vi "pickKeeperRobots.vi"(8 "error in (no error)":errorcluster, 11 "Game in":refnum<class "Game.lvclass">) -> (0 "error out":errorcluster, 3 "Game out":refnum<class "Game.lvclass">)   [LabVIEW 2023, in "Game.lvclass"]
uses:
  Game.lvclass
  Game.lvclass/Game.ctl
  Team_class/Team.lvclass/Team.ctl
  Referee_class/Referee.lvclass/Referee.ctl
  Playbook_class/Playbook.lvclass/Playbook.ctl
  TestPlay_class/TestPlay.lvclass/TestPlay.ctl
  Robot_class/roles.ctl
  Robot_class/Robot.lvclass/Robot.ctl
  Role_class/Role.lvclass/Role.ctl
  HaltPlay_class/HaltPlay.lvclass/HaltPlay.ctl
  TimeoutPlay_class/TimeoutPlay.lvclass/TimeoutPlay.ctl
  ZigZagPlay_class/ZigZagPlay.lvclass/ZigZagPlay.ctl
  Role_class/Write RobotRef.vi
  TestPlay_class/Read Roles.vi
  Robot_class/Write role.vi
  TestPlay_class/Write Roles.vi
  Playbook_class/Write keeper_plays.vi
  Playbook_class/Read keeper_plays.vi
  TestPlay_class/Read NumberOfRobots.vi
  HaltPlay_class/Read Roles.vi
  HaltPlay_class/Write Roles.vi
  HaltPlay_class/Read NumberOfRobots.vi
  TimeoutPlay_class/Read Roles.vi
  TimeoutPlay_class/Write Roles.vi
  ZigZagPlay_class/Read Roles.vi
  ZigZagPlay_class/Write Roles.vi
  Read KeeperTeam.vi
  Read AllyRef.vi
  Read Referee.vi
  Read TestMode IDs.vi
  Referee_class/Read our_goalie_id.vi
  Team_class/Read KeeperPlay.vi
  Team_class/Read RobotRef.vi
  Team_class/Write RobotRef.vi
  Write KeeperTeam.vi
  Ally_class/Ally.lvclass
  C:/Users/roboi/Downloads/VSS_AI-Larc2023/Team_class/Team.lvclass
  TestRole_class/TestRole.lvclass
  C:/Users/roboi/Downloads/VSS_AI-Larc2023/Role_class/Role.lvclass
  HaltRole_class/HaltRole.lvclass
  TimeoutRole_class/TimeoutRole.lvclass
  KeeperRole_class/KeeperRole.lvclass
  ZigZagRole_class/ZigZagRole.lvclass
  Referee_class/Referee.lvclass
  Playbook_class/Playbook.lvclass
  Robot_class/Robot.lvclass
  Play_class/Play.lvclass
  TestPlay_class/TestPlay.lvclass
  HaltPlay_class/HaltPlay.lvclass
  KeeperPlay_class/KeeperPlay.lvclass
  TimeoutPlay_class/TimeoutPlay.lvclass
  ZigZagPlay_class/ZigZagPlay.lvclass
  GoToPlay_class/GoToPlay.lvclass
  Role_class/Role.lvclass
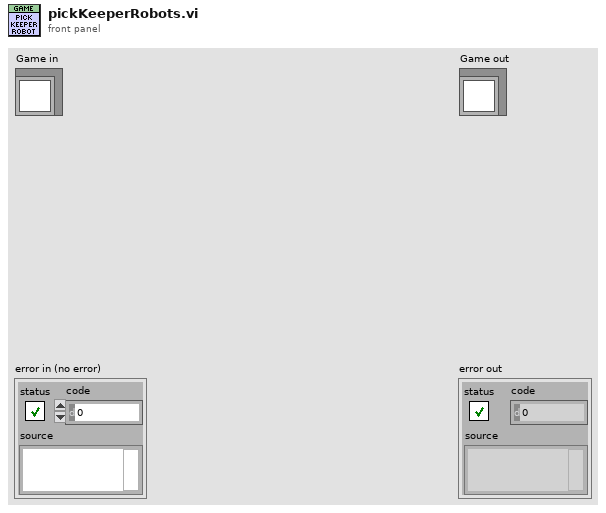
[diagram p1: front panel]
types:
  T1 = typedef "roles.ctl" = enum16{"BallChallengerAttackerVSS", "NormalAttackerVSS", "AttackerAimGoalVSS", "DefenderAreaVSS", "KeeperVSS", "Tabler", "TableFinalizer", "PrepareRollToPassRoller", "PrepareRollToPassReceiver", "SimplePassRoll", "SimplePassRollReceiver", "PenaltyDefense", "PreparePassReceiver 2", "PreparePassReceiver 1", "PassObserver", "Timeout", "Goto", "ZigZag", "None", "BallOutOfField", "DefenderArea", "Duelist", "AttackerStop", "FollowAttacker", "KeeperRole", "KickPenalty", "AttackerAimGoal", "AttackerBlock", "Marker", "Halt", "Shoot", "PassKicker", "PassReceiver", "TestRole", "PenaltyAttacker"}
  T2 = typedef "KeeperPlay.ctl" = enum16{"ZigZag", "Goto", "NormalGame", "KeeperPlay", "Halt", "Timeout", "PenaltyEnemy", "TestPlay"}
  T3 = typedef "keeper_plays.ctl" = cluster{"Play":refnum<class "Play.lvclass">, "TestPlay":refnum<class "TestPlay.lvclass">, "HaltPlay":refnum<class "HaltPlay.lvclass">, "KeeperPlay":refnum<class "KeeperPlay.lvclass">, "TimeoutPlay":refnum<class "TimeoutPlay.lvclass">, "ZigZagPlay":refnum<class "ZigZagPlay.lvclass">, "GoToPlay":refnum<class "GoToPlay.lvclass">}
  T4 = cluster{"TestRole 1":refnum<class "TestRole.lvclass">, "Role":refnum<class "Role.lvclass">, "TestRole 2":refnum<class "TestRole.lvclass">, "TestRole 3":refnum<class "TestRole.lvclass">}
  T5 = cluster{"HaltRole 1":refnum<class "HaltRole.lvclass">, "HaltRole 2":refnum<class "HaltRole.lvclass">, "HaltRole 3":refnum<class "HaltRole.lvclass">, "HaltRole 4":refnum<class "HaltRole.lvclass">, "HaltRole 5":refnum<class "HaltRole.lvclass">, "HaltRole 6":refnum<class "HaltRole.lvclass">}
  T6 = cluster{"TimeoutRole 1":refnum<class "TimeoutRole.lvclass">, "TimeoutRole 2":refnum<class "TimeoutRole.lvclass">, "TimeoutRole 3":refnum<class "TimeoutRole.lvclass">, "TimeoutRole 4":refnum<class "TimeoutRole.lvclass">, "TimeoutRole 5":refnum<class "TimeoutRole.lvclass">, "TimeoutRole 6":refnum<class "TimeoutRole.lvclass">}
  T7 = cluster{"KeeperRole":refnum<class "KeeperRole.lvclass">}
  T8 = cluster{"ZigZagRole":refnum<class "ZigZagRole.lvclass">}
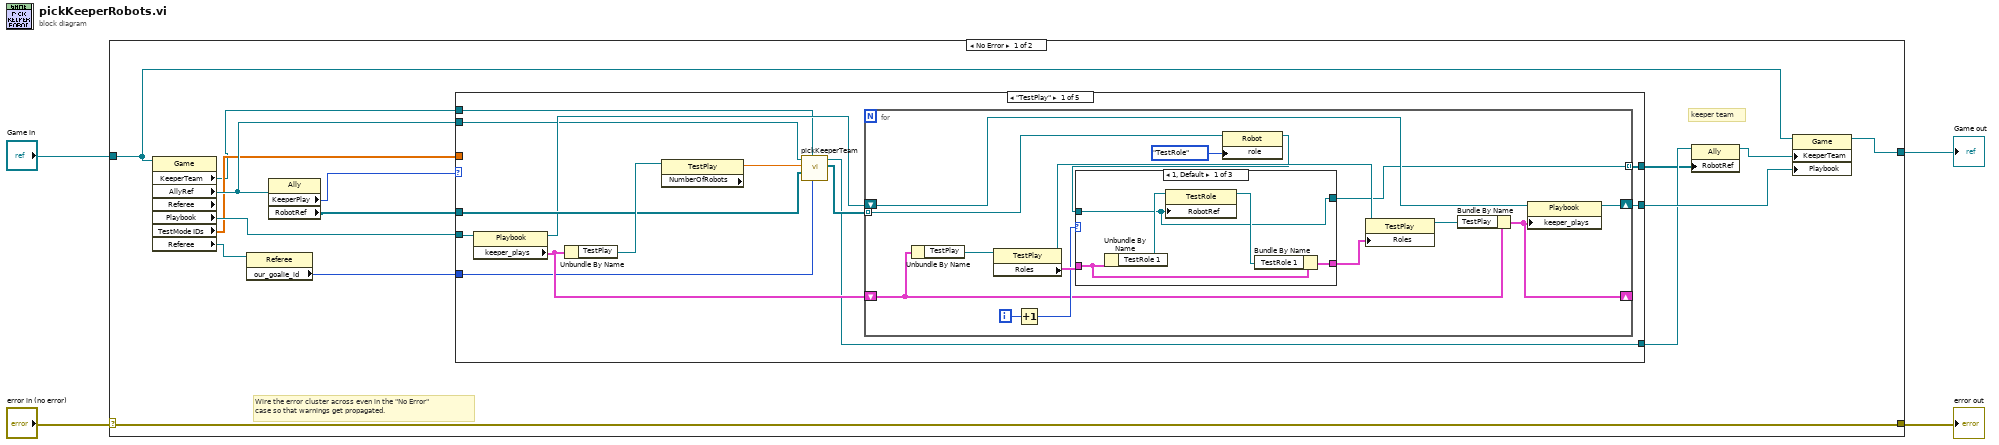
[diagram p0: block diagram]
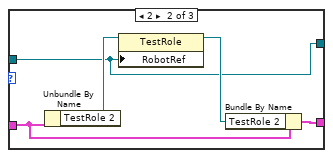
[diagram p2: hidden frame]
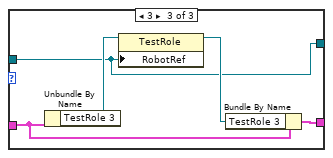
[diagram p3: hidden frame]
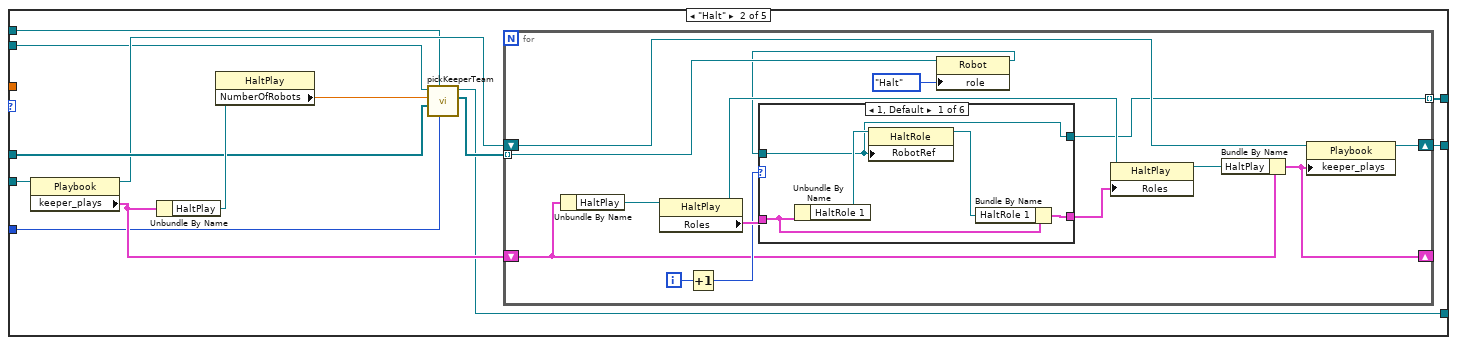
[diagram p4: hidden frame]
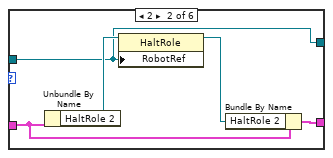
[diagram p5: hidden frame]
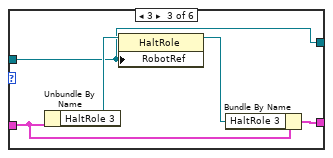
[diagram p6: hidden frame]
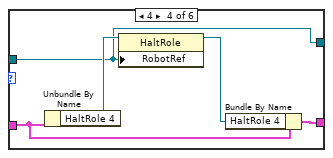
[diagram p7: hidden frame]
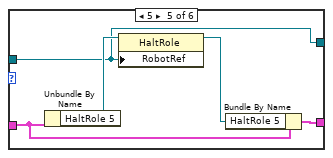
[diagram p8: hidden frame]
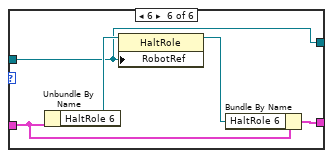
[diagram p9: hidden frame]
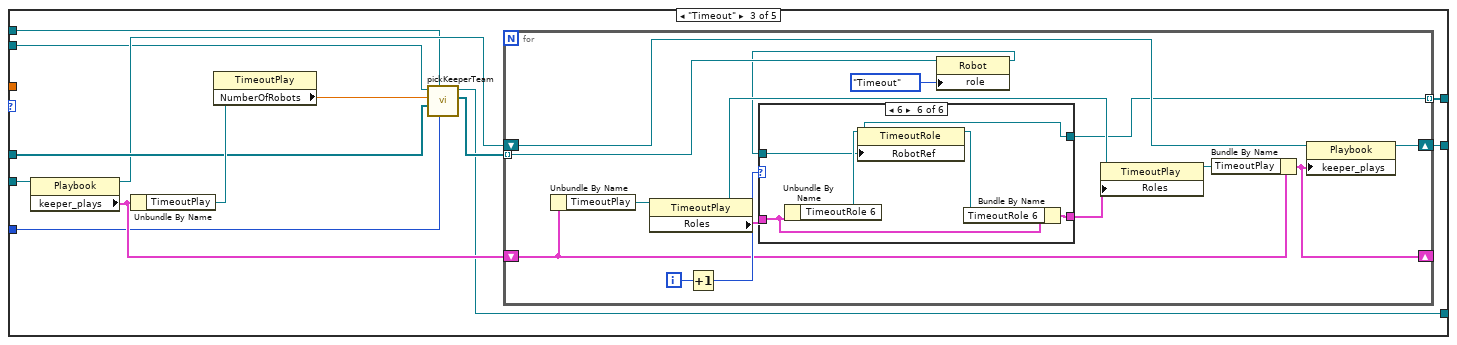
[diagram p10: hidden frame]
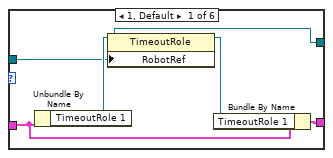
[diagram p11: hidden frame]
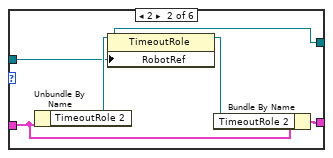
[diagram p12: hidden frame]
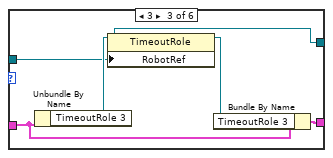
[diagram p13: hidden frame]
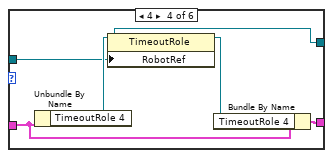
[diagram p14: hidden frame]
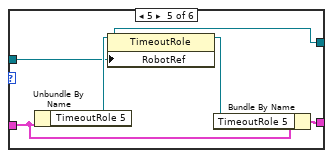
[diagram p15: hidden frame]
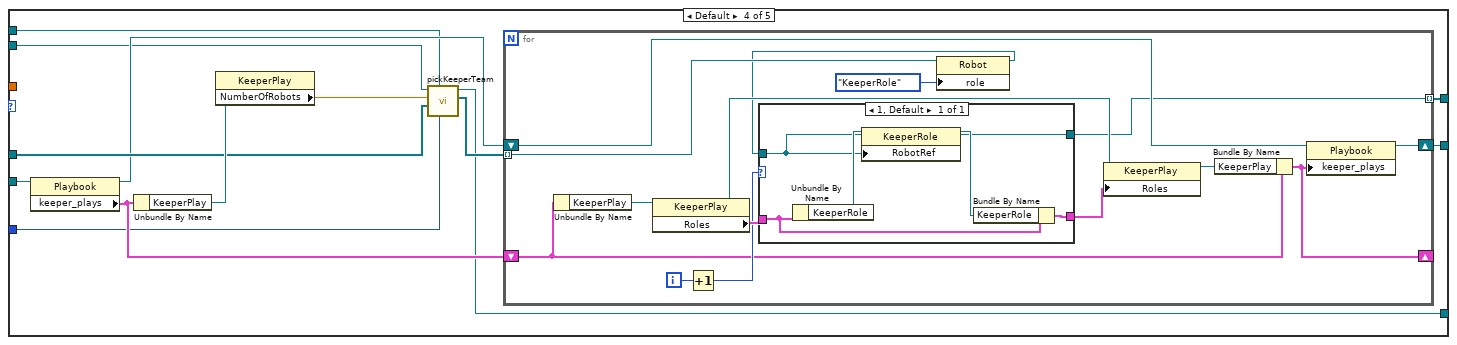
[diagram p16: hidden frame]
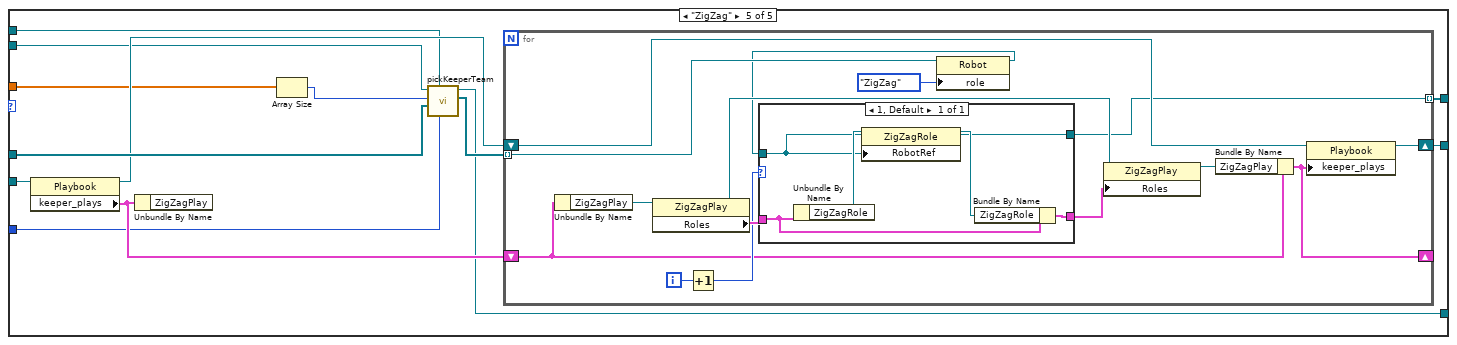
[diagram p17: hidden frame]
diagram:
  n1 = case shown="No Error" "error in (no error)" {
    selector: "error in (no error)" -> [w14 w246]
    tunnel: [w14 w246] -> w3
    tunnel: [w15 w245] -> w1
    tunnel: "Game in" -> [w17 w245]
    frame No Error {
      # "keeper team"
      # "Wire the error cluster across even in the \"No Error\"\ncase so that warnings get propagated."
      n2 = property class="Game" props=["KeeperTeam", "AllyRef", "Referee", "Playbook", "TestMode IDs", "Referee"](reference=w17) -> ("KeeperTeam"=w5:refnum<class "Ally.lvclass">, "AllyRef"=w11:refnum<class "Ally.lvclass">, "Playbook"=w19:refnum<class "Playbook.lvclass">, "TestMode IDs"=w8:dbl[], "Referee"=w7:refnum<class "Referee.lvclass">)  [unwired: 1 in, 3 out]
      n3 = property class="Referee"(reference=w7) -> ("our_goalie_id"=w6:i32)  [unwired: 1 in, 2 out]
      n4 = property class="Ally"(reference=w11) -> ("KeeperPlay"=w9:T2, "RobotRef"=w18:refnum<class "Robot.lvclass">[])  [unwired: 1 in, 2 out]
      n5 = case shown="\"TestPlay\"" w9 {
        tunnel: w19 -> [w32 w75 w133 w191 w224]
        tunnel: w18 -> [w26 w69 w127 w185 w220]
        tunnel: [w30 w73 w131 w189 w222] -> w16
        tunnel: [w29 w72 w130 w188 w221] -> w10
        tunnel: [w23 w66 w124 w182 w217] -> w12
        tunnel: w11 -> [w22 w65 w123 w181 w216]
        tunnel: w8 -> [_ _ _ _ w215]
        tunnel: w6 -> [w21 w64 w122 w180 w213]
        tunnel: w5 -> [w20 w63 w121 w179 w212]
        frame "TestPlay" {
          n6 = property class="Playbook"(reference=w32) -> (reference out=w25:refnum<class "Playbook.lvclass">, "keeper_plays"=w31:T3)  [unwired: 1 in, 1 out]
          n7 = Unbundle By Name(w31) -> ("TestPlay"=w28:refnum<class "TestPlay.lvclass">)
          n8 = property class="TestPlay"(reference=w28) -> ("NumberOfRobots"=w27:dbl)  [unwired: 1 in, 2 out]
          n9 = call-dynamic "pickKeeperTeam.vi"("our_goalie_id"=w21, "OldKepperTeam"=w20, "RobotRef"=w26, "NumberOfRobots"=w27, "Ally in"=w22) -> ("RobotRef out"=w24:refnum<class "Robot.lvclass">[], "Ally out"=w23:refnum<class "Ally.lvclass">)  [unwired: 4 in, 1 out]
          n10 = for {
            tunnel: [w33] -> w29 mode=indexing
            tunnel: w24 -> [w40] mode=indexing
            shift-right: [w42] -> w30
            shift-left: w25 -> [w43]
            shift-right: [w37] -> _
            shift-left: w31 -> [w36]
            i -> [w39]
            n11 = Unbundle By Name(w36) -> ("TestPlay"=w35:refnum<class "TestPlay.lvclass">)
            n12 = property class="TestPlay"(reference=w35) -> (reference out=w45:refnum<class "TestPlay.lvclass">, "Roles"=w47:T4)  [unwired: 1 in, 1 out]
            n13 = Increment(x=w39) -> (x+1=w38:i32)
            n14 = property class="Robot"(reference=w40, "role"=roles."TestRole") -> (reference out=w34:refnum<class "Robot.lvclass">)  [unwired: 1 in, 1 out]
            n15 = case shown="1, Default" w38 {
              tunnel: w47 -> [w51 w56 w61]
              tunnel: [w50 w55 w60] -> w46
              tunnel: w34 -> [w48 w53 w58]
              tunnel: [w48 w53 w58] -> w33
              frame 1, Default {
                n16 = Unbundle By Name(w51) -> ("TestRole 1"=w52:refnum<class "TestRole.lvclass">)
                n17 = property class="TestRole"(reference=w52, "RobotRef"=w48) -> (reference out=w49:refnum<class "TestRole.lvclass">)  [unwired: 1 in, 1 out]
                n18 = Bundle By Name(cluster=w51, "TestRole 1"=w49) -> (w50:T4)
              }
              frame 2 {
                n19 = Unbundle By Name(w56) -> ("TestRole 2"=w57:refnum<class "TestRole.lvclass">)
                n20 = property class="TestRole"(reference=w57, "RobotRef"=w53) -> (reference out=w54:refnum<class "TestRole.lvclass">)  [unwired: 1 in, 1 out]
                n21 = Bundle By Name(cluster=w56, "TestRole 2"=w54) -> (w55:T4)
              }
              frame 3 {
                n22 = Unbundle By Name(w61) -> ("TestRole 3"=w62:refnum<class "TestRole.lvclass">)
                n23 = property class="TestRole"(reference=w62, "RobotRef"=w58) -> (reference out=w59:refnum<class "TestRole.lvclass">)  [unwired: 1 in, 1 out]
                n24 = Bundle By Name(cluster=w61, "TestRole 3"=w59) -> (w60:T4)
              }
            }
            n25 = property class="TestPlay"(reference=w45, "Roles"=w46) -> (reference out=w44:refnum<class "TestPlay.lvclass">)  [unwired: 1 in, 1 out]
            n26 = Bundle By Name(cluster=w36, "TestPlay"=w44) -> (w37:T3)
            n27 = property class="Playbook"(reference=w43, "keeper_plays"=w37) -> (reference out=w42:refnum<class "Playbook.lvclass">)  [unwired: 1 in, 1 out]
          }
        }
        frame "Halt" {
          n28 = property class="Playbook"(reference=w75) -> (reference out=w68:refnum<class "Playbook.lvclass">, "keeper_plays"=w74:T3)  [unwired: 1 in, 1 out]
          n29 = Unbundle By Name(w74) -> ("HaltPlay"=w71:refnum<class "HaltPlay.lvclass">)
          n30 = property class="HaltPlay"(reference=w71) -> ("NumberOfRobots"=w70:dbl)  [unwired: 1 in, 2 out]
          n31 = call-dynamic "pickKeeperTeam.vi"("our_goalie_id"=w64, "OldKepperTeam"=w63, "RobotRef"=w69, "NumberOfRobots"=w70, "Ally in"=w65) -> ("RobotRef out"=w67:refnum<class "Robot.lvclass">[], "Ally out"=w66:refnum<class "Ally.lvclass">)  [unwired: 4 in, 1 out]
          n32 = for {
            tunnel: [w77] -> w72 mode=indexing
            tunnel: w67 -> [w83] mode=indexing
            shift-right: [w85] -> w73
            shift-left: w68 -> [w86]
            shift-right: [w80] -> _
            shift-left: w74 -> [w79]
            i -> [w82]
            n33 = Unbundle By Name(w79) -> ("HaltPlay"=w78:refnum<class "HaltPlay.lvclass">)
            n34 = property class="HaltPlay"(reference=w78) -> (reference out=w88:refnum<class "HaltPlay.lvclass">, "Roles"=w90:T5)  [unwired: 1 in, 1 out]
            n35 = Increment(x=w82) -> (x+1=w81:i32)
            n36 = property class="Robot"(reference=w83, "role"=roles."Halt") -> (reference out=w76:refnum<class "Robot.lvclass">)  [unwired: 1 in, 1 out]
            n37 = case shown="1, Default" w81 {
              tunnel: w90 -> [w94 w99 w104 w109 w114 w119]
              tunnel: [w93 w98 w103 w108 w113 w118] -> w89
              tunnel: w76 -> [w91 w96 w101 w106 w111 w116]
              tunnel: [w91 w96 w101 w106 w111 w116] -> w77
              frame 1, Default {
                n38 = Unbundle By Name(w94) -> ("HaltRole 1"=w95:refnum<class "HaltRole.lvclass">)
                n39 = property class="HaltRole"(reference=w95, "RobotRef"=w91) -> (reference out=w92:refnum<class "HaltRole.lvclass">)  [unwired: 1 in, 1 out]
                n40 = Bundle By Name(cluster=w94, "HaltRole 1"=w92) -> (w93:T5)
              }
              frame 2 {
                n41 = Unbundle By Name(w99) -> ("HaltRole 2"=w100:refnum<class "HaltRole.lvclass">)
                n42 = property class="HaltRole"(reference=w100, "RobotRef"=w96) -> (reference out=w97:refnum<class "HaltRole.lvclass">)  [unwired: 1 in, 1 out]
                n43 = Bundle By Name(cluster=w99, "HaltRole 2"=w97) -> (w98:T5)
              }
              frame 3 {
                n44 = Unbundle By Name(w104) -> ("HaltRole 3"=w105:refnum<class "HaltRole.lvclass">)
                n45 = property class="HaltRole"(reference=w105, "RobotRef"=w101) -> (reference out=w102:refnum<class "HaltRole.lvclass">)  [unwired: 1 in, 1 out]
                n46 = Bundle By Name(cluster=w104, "HaltRole 3"=w102) -> (w103:T5)
              }
              frame 4 {
                n47 = Unbundle By Name(w109) -> ("HaltRole 4"=w110:refnum<class "HaltRole.lvclass">)
                n48 = property class="HaltRole"(reference=w110, "RobotRef"=w106) -> (reference out=w107:refnum<class "HaltRole.lvclass">)  [unwired: 1 in, 1 out]
                n49 = Bundle By Name(cluster=w109, "HaltRole 4"=w107) -> (w108:T5)
              }
              frame 5 {
                n50 = Unbundle By Name(w114) -> ("HaltRole 5"=w115:refnum<class "HaltRole.lvclass">)
                n51 = property class="HaltRole"(reference=w115, "RobotRef"=w111) -> (reference out=w112:refnum<class "HaltRole.lvclass">)  [unwired: 1 in, 1 out]
                n52 = Bundle By Name(cluster=w114, "HaltRole 5"=w112) -> (w113:T5)
              }
              frame 6 {
                n53 = Unbundle By Name(w119) -> ("HaltRole 6"=w120:refnum<class "HaltRole.lvclass">)
                n54 = property class="HaltRole"(reference=w120, "RobotRef"=w116) -> (reference out=w117:refnum<class "HaltRole.lvclass">)  [unwired: 1 in, 1 out]
                n55 = Bundle By Name(cluster=w119, "HaltRole 6"=w117) -> (w118:T5)
              }
            }
            n56 = property class="HaltPlay"(reference=w88, "Roles"=w89) -> (reference out=w87:refnum<class "HaltPlay.lvclass">)  [unwired: 1 in, 1 out]
            n57 = Bundle By Name(cluster=w79, "HaltPlay"=w87) -> (w80:T3)
            n58 = property class="Playbook"(reference=w86, "keeper_plays"=w80) -> (reference out=w85:refnum<class "Playbook.lvclass">)  [unwired: 1 in, 1 out]
          }
        }
        frame "Timeout" {
          n59 = property class="Playbook"(reference=w133) -> (reference out=w126:refnum<class "Playbook.lvclass">, "keeper_plays"=w132:T3)  [unwired: 1 in, 1 out]
          n60 = Unbundle By Name(w132) -> ("TimeoutPlay"=w129:refnum<class "TimeoutPlay.lvclass">)
          n61 = property class="TimeoutPlay"(reference=w129) -> ("NumberOfRobots"=w128:dbl)  [unwired: 1 in, 2 out]
          n62 = call-dynamic "pickKeeperTeam.vi"("our_goalie_id"=w122, "OldKepperTeam"=w121, "RobotRef"=w127, "NumberOfRobots"=w128, "Ally in"=w123) -> ("RobotRef out"=w125:refnum<class "Robot.lvclass">[], "Ally out"=w124:refnum<class "Ally.lvclass">)  [unwired: 4 in, 1 out]
          n63 = for {
            tunnel: [w135] -> w130 mode=indexing
            tunnel: w125 -> [w141] mode=indexing
            shift-right: [w143] -> w131
            shift-left: w126 -> [w144]
            shift-right: [w138] -> _
            shift-left: w132 -> [w137]
            i -> [w140]
            n64 = Unbundle By Name(w137) -> ("TimeoutPlay"=w136:refnum<class "TimeoutPlay.lvclass">)
            n65 = property class="TimeoutPlay"(reference=w136) -> (reference out=w146:refnum<class "TimeoutPlay.lvclass">, "Roles"=w148:T6)  [unwired: 1 in, 1 out]
            n66 = Increment(x=w140) -> (x+1=w139:i32)
            n67 = property class="Robot"(reference=w141, "role"=roles."Timeout") -> (reference out=w134:refnum<class "Robot.lvclass">)  [unwired: 1 in, 1 out]
            n68 = case shown="6" w139 {
              tunnel: w148 -> [w152 w157 w162 w167 w172 w177]
              tunnel: [w151 w156 w161 w166 w171 w176] -> w147
              tunnel: w134 -> [w149 w154 w159 w164 w169 w174]
              tunnel: [w149 w154 w159 w164 w169 w174] -> w135
              frame 1, Default {
                n69 = Unbundle By Name(w152) -> ("TimeoutRole 1"=w153:refnum<class "TimeoutRole.lvclass">)
                n70 = property class="TimeoutRole"(reference=w153, "RobotRef"=w149) -> (reference out=w150:refnum<class "TimeoutRole.lvclass">)  [unwired: 1 in, 1 out]
                n71 = Bundle By Name(cluster=w152, "TimeoutRole 1"=w150) -> (w151:T6)
              }
              frame 2 {
                n72 = Unbundle By Name(w157) -> ("TimeoutRole 2"=w158:refnum<class "TimeoutRole.lvclass">)
                n73 = property class="TimeoutRole"(reference=w158, "RobotRef"=w154) -> (reference out=w155:refnum<class "TimeoutRole.lvclass">)  [unwired: 1 in, 1 out]
                n74 = Bundle By Name(cluster=w157, "TimeoutRole 2"=w155) -> (w156:T6)
              }
              frame 3 {
                n75 = Unbundle By Name(w162) -> ("TimeoutRole 3"=w163:refnum<class "TimeoutRole.lvclass">)
                n76 = property class="TimeoutRole"(reference=w163, "RobotRef"=w159) -> (reference out=w160:refnum<class "TimeoutRole.lvclass">)  [unwired: 1 in, 1 out]
                n77 = Bundle By Name(cluster=w162, "TimeoutRole 3"=w160) -> (w161:T6)
              }
              frame 4 {
                n78 = Unbundle By Name(w167) -> ("TimeoutRole 4"=w168:refnum<class "TimeoutRole.lvclass">)
                n79 = property class="TimeoutRole"(reference=w168, "RobotRef"=w164) -> (reference out=w165:refnum<class "TimeoutRole.lvclass">)  [unwired: 1 in, 1 out]
                n80 = Bundle By Name(cluster=w167, "TimeoutRole 4"=w165) -> (w166:T6)
              }
              frame 5 {
                n81 = Unbundle By Name(w172) -> ("TimeoutRole 5"=w173:refnum<class "TimeoutRole.lvclass">)
                n82 = property class="TimeoutRole"(reference=w173, "RobotRef"=w169) -> (reference out=w170:refnum<class "TimeoutRole.lvclass">)  [unwired: 1 in, 1 out]
                n83 = Bundle By Name(cluster=w172, "TimeoutRole 5"=w170) -> (w171:T6)
              }
              frame 6 {
                n84 = Unbundle By Name(w177) -> ("TimeoutRole 6"=w178:refnum<class "TimeoutRole.lvclass">)
                n85 = property class="TimeoutRole"(reference=w178, "RobotRef"=w174) -> (reference out=w175:refnum<class "TimeoutRole.lvclass">)  [unwired: 1 in, 1 out]
                n86 = Bundle By Name(cluster=w177, "TimeoutRole 6"=w175) -> (w176:T6)
              }
            }
            n87 = property class="TimeoutPlay"(reference=w146, "Roles"=w147) -> (reference out=w145:refnum<class "TimeoutPlay.lvclass">)  [unwired: 1 in, 1 out]
            n88 = Bundle By Name(cluster=w137, "TimeoutPlay"=w145) -> (w138:T3)
            n89 = property class="Playbook"(reference=w144, "keeper_plays"=w138) -> (reference out=w143:refnum<class "Playbook.lvclass">)  [unwired: 1 in, 1 out]
          }
        }
        frame Default {
          n90 = property class="Playbook"(reference=w191) -> (reference out=w184:refnum<class "Playbook.lvclass">, "keeper_plays"=w190:T3)  [unwired: 1 in, 1 out]
          n91 = Unbundle By Name(w190) -> ("KeeperPlay"=w187:refnum<class "KeeperPlay.lvclass">)
          n92 = property class="KeeperPlay"(reference=w187) -> ("NumberOfRobots"=w186:dbl)  [unwired: 1 in, 2 out]
          n93 = call-dynamic "pickKeeperTeam.vi"("our_goalie_id"=w180, "OldKepperTeam"=w179, "RobotRef"=w185, "NumberOfRobots"=w186, "Ally in"=w181) -> ("RobotRef out"=w183:refnum<class "Robot.lvclass">[], "Ally out"=w182:refnum<class "Ally.lvclass">)  [unwired: 4 in, 1 out]
          n94 = for {
            tunnel: [w192] -> w188 mode=indexing
            tunnel: w183 -> [w199] mode=indexing
            shift-right: [w201] -> w189
            shift-left: w184 -> [w202]
            shift-right: [w196] -> _
            shift-left: w190 -> [w195]
            i -> [w198]
            n95 = Unbundle By Name(w195) -> ("KeeperPlay"=w194:refnum<class "KeeperPlay.lvclass">)
            n96 = property class="KeeperPlay"(reference=w194) -> (reference out=w204:refnum<class "KeeperPlay.lvclass">, "Roles"=w206:T7)  [unwired: 1 in, 1 out]
            n97 = Increment(x=w198) -> (x+1=w197:i32)
            n98 = property class="Robot"(reference=w199, "role"=roles."KeeperRole") -> (reference out=w193:refnum<class "Robot.lvclass">)  [unwired: 1 in, 1 out]
            n99 = case shown="1, Default" w197 {
              tunnel: w206 -> [w210]
              tunnel: [w209] -> w205
              tunnel: w193 -> [w207]
              tunnel: [w207] -> w192
              frame 1, Default {
                n100 = Unbundle By Name(w210) -> ("KeeperRole"=w211:refnum<class "KeeperRole.lvclass">)
                n101 = property class="KeeperRole"(reference=w211, "RobotRef"=w207) -> (reference out=w208:refnum<class "KeeperRole.lvclass">)  [unwired: 1 in, 1 out]
                n102 = Bundle By Name(cluster=w210, "KeeperRole"=w208) -> (w209:T7)
              }
            }
            n103 = property class="KeeperPlay"(reference=w204, "Roles"=w205) -> (reference out=w203:refnum<class "KeeperPlay.lvclass">)  [unwired: 1 in, 1 out]
            n104 = Bundle By Name(cluster=w195, "KeeperPlay"=w203) -> (w196:T3)
            n105 = property class="Playbook"(reference=w202, "keeper_plays"=w196) -> (reference out=w201:refnum<class "Playbook.lvclass">)  [unwired: 1 in, 1 out]
          }
        }
        frame "ZigZag" {
          n106 = property class="Playbook"(reference=w224) -> (reference out=w219:refnum<class "Playbook.lvclass">, "keeper_plays"=w223:T3)  [unwired: 1 in, 1 out]
          n107 = Unbundle By Name(w223) -> ()  [unwired: 1 out]
          n108 = Array Size(array=w215) -> (size(s)=w214:i32)
          n109 = call-dynamic "pickKeeperTeam.vi"("our_goalie_id"=w213, "OldKepperTeam"=w212, "RobotRef"=w220, "NumberOfRobots"=w214, "Ally in"=w216) -> ("RobotRef out"=w218:refnum<class "Robot.lvclass">[], "Ally out"=w217:refnum<class "Ally.lvclass">)  [unwired: 4 in, 1 out]
          n110 = for {
            tunnel: [w225] -> w221 mode=indexing
            tunnel: w218 -> [w232] mode=indexing
            shift-right: [w234] -> w222
            shift-left: w219 -> [w235]
            shift-right: [w229] -> _
            shift-left: w223 -> [w228]
            i -> [w231]
            n111 = Unbundle By Name(w228) -> ("ZigZagPlay"=w227:refnum<class "ZigZagPlay.lvclass">)
            n112 = property class="ZigZagPlay"(reference=w227) -> (reference out=w237:refnum<class "ZigZagPlay.lvclass">, "Roles"=w239:T8)  [unwired: 1 in, 1 out]
            n113 = Increment(x=w231) -> (x+1=w230:i32)
            n114 = property class="Robot"(reference=w232, "role"=roles."ZigZag") -> (reference out=w226:refnum<class "Robot.lvclass">)  [unwired: 1 in, 1 out]
            n115 = case shown="1, Default" w230 {
              tunnel: w239 -> [w243]
              tunnel: [w242] -> w238
              tunnel: w226 -> [w240]
              tunnel: [w240] -> w225
              frame 1, Default {
                n116 = Unbundle By Name(w243) -> ("ZigZagRole"=w244:refnum<class "ZigZagRole.lvclass">)
                n117 = property class="ZigZagRole"(reference=w244, "RobotRef"=w240) -> (reference out=w241:refnum<class "ZigZagRole.lvclass">)  [unwired: 1 in, 1 out]
                n118 = Bundle By Name(cluster=w243, "ZigZagRole"=w241) -> (w242:T8)
              }
            }
            n119 = property class="ZigZagPlay"(reference=w237, "Roles"=w238) -> (reference out=w236:refnum<class "ZigZagPlay.lvclass">)  [unwired: 1 in, 1 out]
            n120 = Bundle By Name(cluster=w228, "ZigZagPlay"=w236) -> (w229:T3)
            n121 = property class="Playbook"(reference=w235, "keeper_plays"=w229) -> (reference out=w234:refnum<class "Playbook.lvclass">)  [unwired: 1 in, 1 out]
          }
        }
      }
      n122 = property class="Ally"(reference=w12, "RobotRef"=w10) -> (reference out=w13:refnum<class "Ally.lvclass">)  [unwired: 1 in, 1 out]
      n123 = property class="Game"(reference=w17, "KeeperTeam"=w13, "Playbook"=w16) -> (reference out=w15:refnum<class "Game.lvclass">)  [unwired: 1 in, 1 out]
    }
    frame Error {
    }
  }
  "error out" <- w3
  "Game out" <- w1
